vi "Horizontal Panel Example.vi"() -> ()   [LabVIEW 2016, in "PanelExample.lvclass"]
uses:
  PanelExample.lvclass
  PanelObject/PanelObject.lvclass
  <vilib>/Utility/error.llb/DialogType.ctl
  PanelDataNode/PanelDataNode.lvclass
  PanelDataNode/PanelDataNode.lvclass/PanelDataNode.ctl
  PanelDataNode/Split Mode.ctl
  QueueManager.llb/CreatQueue.vi
  QueueManager.llb/Remove.vi
  QueueManager.llb/Destroy.vi
  QueueManager.llb/Insert.vi
panel:
  in  "Node*":refnum<data-value>
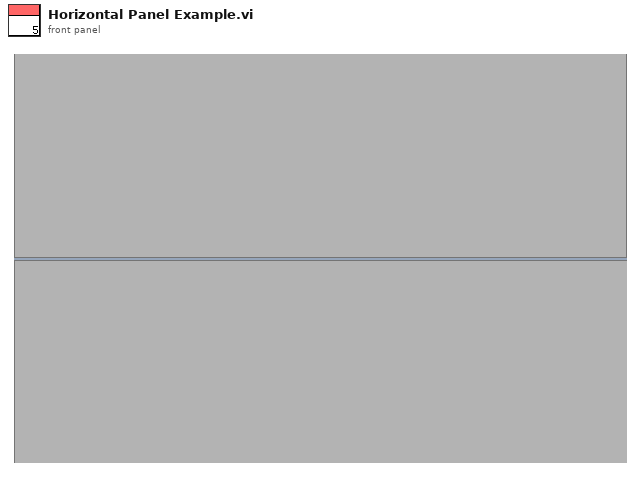
[diagram p1: front panel]
types:
  T1 = cluster{"error":errorcluster, "Event":string, "Data":variant, "Q_Local":string, "Caller":string, "Q_Root":string}
  T2 = typedef "PanelDataNode.lvclass/Split Mode.ctl" = enum16{"Horizontal(up)", "Vertical(left)", "Horizontal(down)", "Vertical(right)"}
  T3 = typedef "DialogType.ctl" = u16
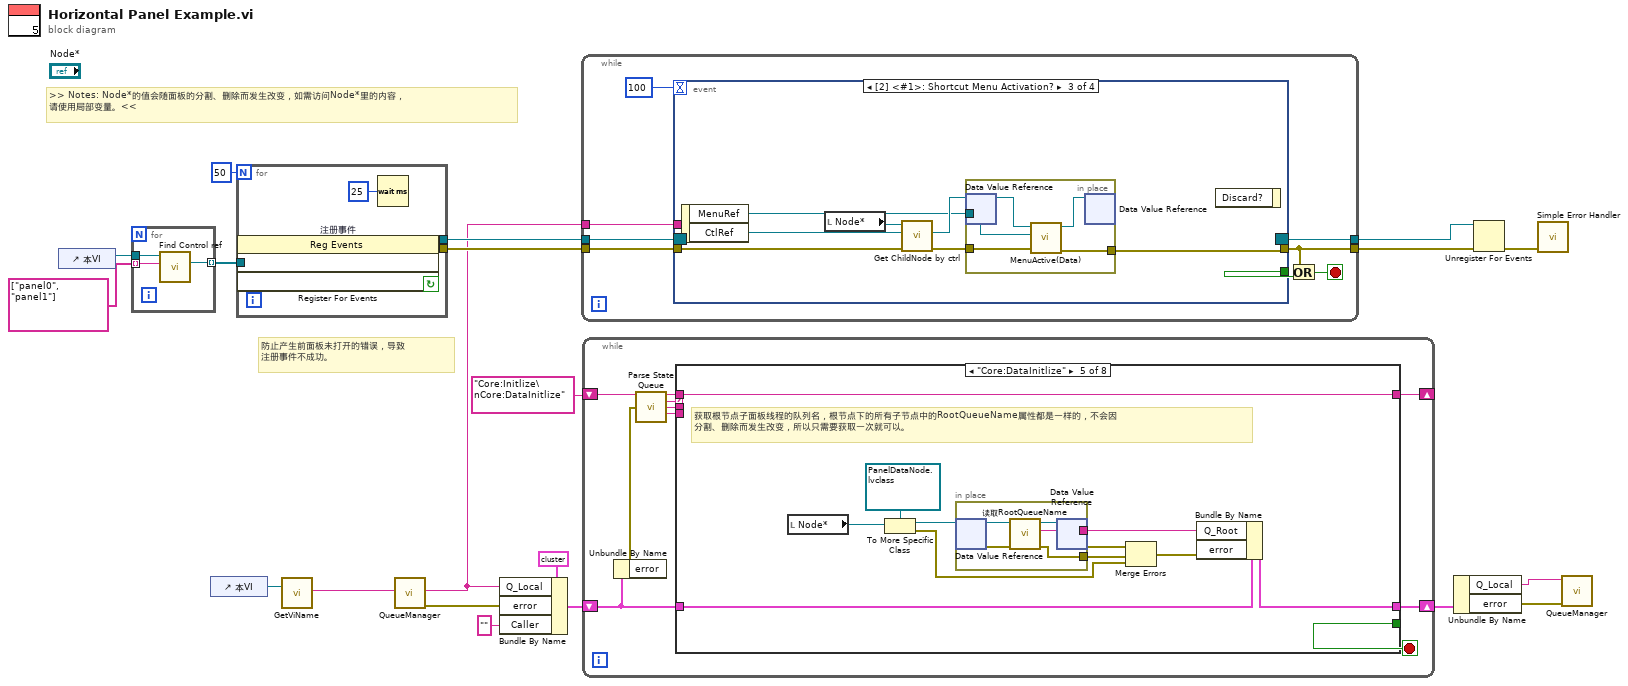
[diagram p0: block diagram]
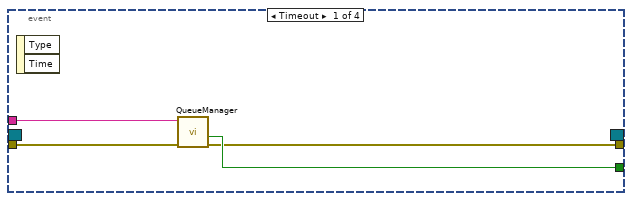
[diagram p2: hidden frame]
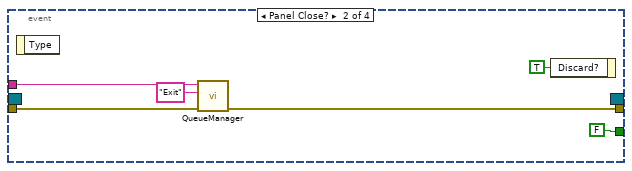
[diagram p3: hidden frame]
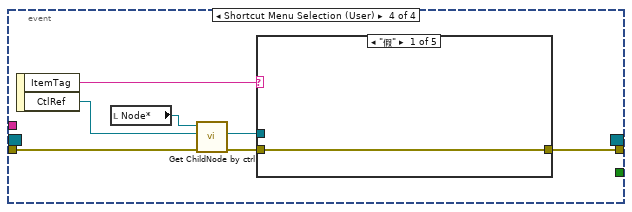
[diagram p4: hidden frame]
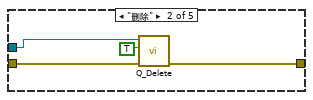
[diagram p5: hidden frame]
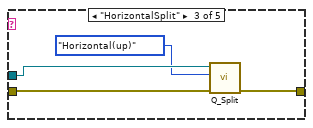
[diagram p6: hidden frame]
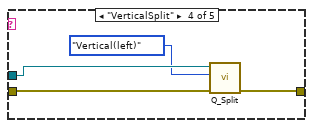
[diagram p7: hidden frame]
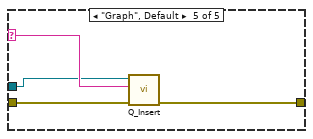
[diagram p8: hidden frame]
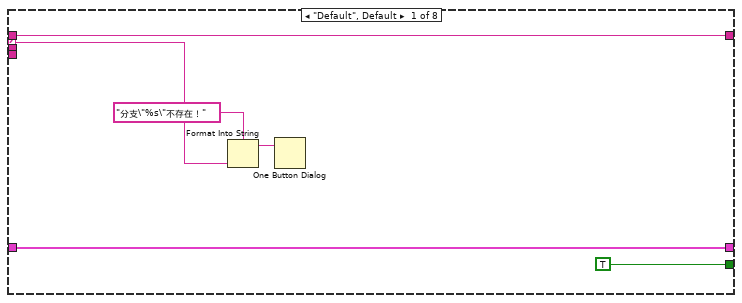
[diagram p9: hidden frame]
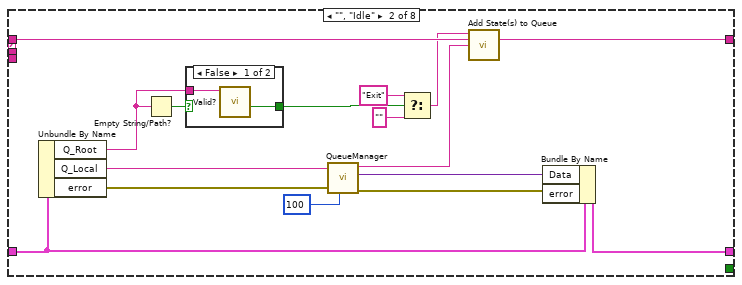
[diagram p10: hidden frame]
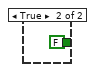
[diagram p11: hidden frame]
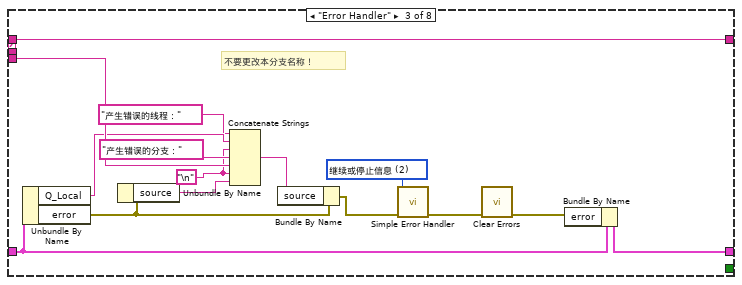
[diagram p12: hidden frame]
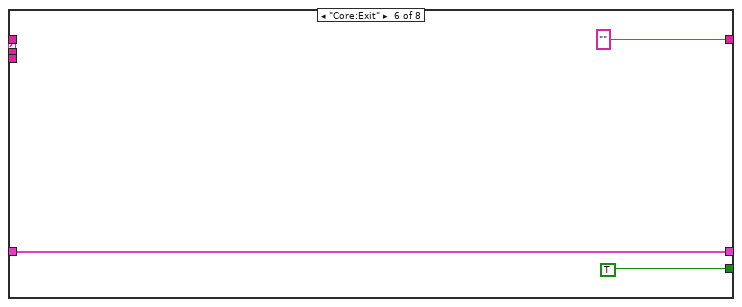
[diagram p14: hidden frame]
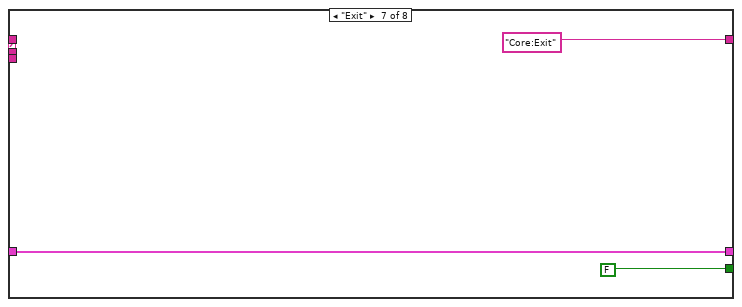
[diagram p15: hidden frame]
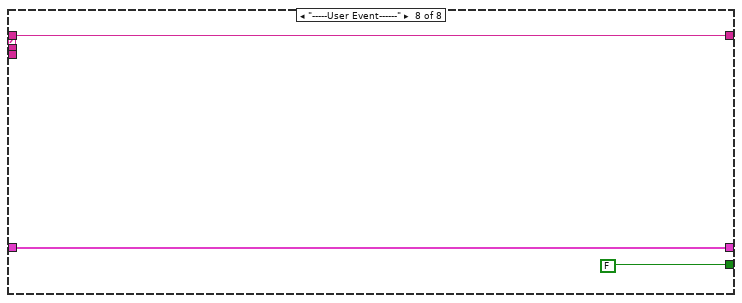
[diagram p16: hidden frame]
diagram:
  # ">> Notes: Node*的值会随面板的分割、删除而发生改变，如需访问Node*里的内容，\n请使用局部变量。<<"
  # "防止产生前面板未打开的错误，导致\n注册事件不成功。"
  n1 = control-ref of="本VI"() -> (w2:refnum<vi>)
  n2 = for {
    tunnel: w2 -> [w22]
    tunnel: string[] ["panel0", "panel1"] -> [w21] mode=indexing
    tunnel: [w20] -> w7 mode=indexing
    n3 = call "Find Control ref.vi"("control name"=w21, "panelvi*"=w22) -> ("ctrl*"=w20:refnum<vi>)  [unwired: 7 in, 2 out]
  }
  n4 = control-ref of="本VI"() -> (w12:refnum<vi>)
  n5 = for {
    N: 50 -> [_]
    tunnel: [w24] -> w10
    tunnel: [w26] -> w9
    tunnel: w7 -> [w25]
    stop <- w24 continue-if-true
    n6 = register-events "注册事件"(w25, w25) -> (reference out=w26:refnum<event-registration>, error out=w24:errorcluster)  [unwired: 2 in]
    n7 = Wait (ms)(milliseconds to wait=u32 25 ("等待时间（毫秒）")) -> ()  [unwired: 1 out]
  }
  n8 = call "GetViName.vi"("VI*"=w12) -> ("VI Name"=w8:string)  [unwired: 9 in, 1 out]
  n9 = call-poly "QueueManager.vi"("QueueName"=w8) -> ("error out"=w11:errorcluster)  [unwired: 9 in, 1 out]
  n10 = Bundle By Name(cluster=T1 {"error"={"status"=FALSE, "code"=0, "source"=""}, "Event"="", "Data"=variant, "Q_Local"="", "Caller"="", "Q_Root"=""} ("TmpData"), "Q_Local"=w8, "error"=w11, "Caller"="") -> (w15:T1)
  n11 = while {
    tunnel: w10 -> [w28]
    tunnel: w8 -> [w34]
    tunnel: [w31] -> w5
    tunnel: w9 -> [w29]
    tunnel: [w27] -> w3
    stop <- w32 stop-if-true
    n12 = event shown="[2] <#1>: Shortcut Menu Activation?" {
      selector: w29 -> [_ _ _ _]
      dyn-events: [_ _ _ _] -> w27
      timeout: 100 -> [_ _ _ _]
      tunnel: [w36 FALSE _ _] -> w33
      tunnel: w34 -> [w38 w43 _ _]
      tunnel: w28 -> [w37 w42 w48 w62]
      tunnel: [w35 w41 w46 w60] -> w31
      event Timeout {
        n13 = event-data() -> ()  [unwired: 1 in, 2 out]
        n14 = call-poly "QueueManager.vi"("error in (no error)"=w37, "Queue Name(unamed)"=w38) -> ("error out"=w35:errorcluster, "Not Exist?"=w36:bool)  [unwired: 8 in]
      }
      event Panel Close? {
        n15 = event-data() -> ()  [unwired: 1 in, 1 out]
        n16 = call-poly "QueueManager.vi"("error in"=w42, "Event"="Exit", "QueueName"=w43) -> ("error out"=w41:errorcluster)  [unwired: 7 in, 1 out]
        n17 = event-data("Discard?"=TRUE ("放弃？")) -> ()  [unwired: 1 in, 1 out]
      }
      event Shortcut Menu Activation? {
        n18 = event-data() -> ("MenuRef"=w45:refnum<k9>, "CtlRef"=w49:refnum<vi>)  [unwired: 1 in]
        n19 = local read "Node*"() -> (w50:refnum<data-value>)
        n20 = call "Get ChildNode by ctrl.vi"("error in (no error)"=w48, "ctr*"=w49, "Node*"=w50) -> ("error out"=w47:errorcluster, "ChildNode*"=w51:refnum<data-value>)  [unwired: 7 in]
        n21 = in-place {
          in-place-border: w45 -> [w55]
          in-place-border: w47 -> [w53]
          in-place-border: [w52] -> w46
          n22 = in-place-dvr #1(w51) -> (w56:refnum<class "PanelDataNode.lvclass">)  [unwired: 1 out]
          n23 = call-dynamic "MenuActive(Data).vi"("error in"=w53, "Menu Reference in"=w55, "PanelDataNode in"=w56) -> ("error out"=w52:errorcluster, "PanelDataNode out"=w54:refnum<class "PanelDataNode.lvclass">)  [unwired: 6 in, 1 out]
          n24 = in-place-dvr #1(w54) -> ()  [unwired: 2 out]
        }
        n25 = event-data() -> ()  [unwired: 2 in, 1 out]
      }
      event Shortcut Menu Selection (User) {
        n26 = event-data() -> ("ItemTag"=w59:string, "CtlRef"=w63:refnum<vi>)  [unwired: 1 in]
        n27 = local read "Node*"() -> (w57:refnum<data-value>)
        n28 = call "Get ChildNode by ctrl.vi"("error in (no error)"=w62, "ctr*"=w63, "Node*"=w57) -> ("error out"=w61:errorcluster, "ChildNode*"=w58:refnum<data-value>)  [unwired: 7 in]
        n29 = case shown="\"假\"" w59 {
          selector: w59 -> [_ _ _ _ w80]
          tunnel: w61 -> [w64 w67 w72 w76 w79]
          tunnel: [w64 w66 w71 w75 w77] -> w60
          tunnel: w58 -> [_ w65 w70 w74 w78]
          frame "假" {
          }
          frame "删除" {
            n30 = call "Q_Delete.vi"("error in"=w67, "CloseVI?(T)"=TRUE, "ChildNode*"=w65) -> ("error out"=w66:errorcluster)  [unwired: 8 in]
          }
          frame "HorizontalSplit" {
            n31 = call "Q_Split.vi"("error in"=w72, "Split Mode"=Split_Mode."Horizontal(up)", "ChildNode*"=w70) -> ("error out"=w71:errorcluster)  [unwired: 8 in]
          }
          frame "VerticalSplit" {
            n32 = call "Q_Split.vi"("error in"=w76, "Split Mode"=Split_Mode."Vertical(left)", "ChildNode*"=w74) -> ("error out"=w75:errorcluster)  [unwired: 8 in]
          }
          frame "Graph", Default {
            n33 = call "Q_Insert.vi"("error in"=w79, "Vi Alias"=w80, "ChildNode*"=w78) -> ("error out"=w77:errorcluster)  [unwired: 8 in]
          }
        }
      }
    }
    n34 = Or(x=w31, y=w33) -> (x .or. y?=w32:bool)
  }
  n35 = while {
    shift-right: [w84] -> w17
    shift-left: w15 -> [w85]
    shift-right: [w83] -> _
    shift-left: "Core:Initlize\nCore:DataInitlize" -> [w90]
    stop <- w87 stop-if-true
    n36 = Unbundle By Name(w85) -> ("error"=w86:errorcluster)
    n37 = call "Parse State Queue.vi"("State Queue"=w90, "Error In (no error)"=w86) -> ("Remaining States"=w89:string, "Current State"=w88:string, "Arguments"=w82:string, "PreState"=w81:string)  [unwired: 10 in]
    n38 = case shown="\"Core:DataInitlize\"" w88 {
      selector: w88 -> [w94 _ _ _ _ _ _ _]
      tunnel: w89 -> [w95 w109 w130 w132 w143 _ _ w155]
      tunnel: w82 -> [_ _ _ _ _ _ _ _]
      tunnel: [TRUE _ _ _ _ TRUE FALSE FALSE] -> w87
      tunnel: w85 -> [w96 w106 w127 w131 w139 w150 w153 w156]
      tunnel: [w96 w111 w126 w131 w138 w150 w153 w156] -> w84
      tunnel: [w95 w108 w130 w132 w143 "" ("Remaining States") "Core:Exit" ("Remaining States") w155] -> w83
      tunnel: w81 -> [_ _ w124 _ _ _ _ _]
      frame "Default", Default {
        n39 = Format Into String(format string="分支\"%s\"不存在！" ("格式字符串"), w94) -> (resulting string=w93:string)  [unwired: 2 in, 1 out]
        n40 = One Button Dialog(message=w93) -> ()  [unwired: 1 in, 1 out]
      }
      frame "", "Idle" {
        n41 = Unbundle By Name(w106) -> ("Q_Root"=w100:string, "Q_Local"=w105:string, "error"=w104:errorcluster)
        n42 = Empty String/Path?(string/path=w100) -> (empty?=w103:bool)
        n43 = case shown="False" w103 {
          tunnel: [w114 FALSE ("Not Exist?")] -> w102
          tunnel: w100 -> [w113 _]
          frame False {
            n44 = call "Valid?.vi"("Queue Name(unamed)"=w113) -> ("Not Exist?"=w114:bool)  [unwired: 9 in, 1 out]
          }
          frame True {
          }
        }
        n45 = call-poly "QueueManager.vi"("Time out(-1)"=100, "error in (no error)"=w104, "Queue Name"=w105) -> ("error out"=w112:errorcluster, "Data"=w110:variant, "Event"=w99:string)  [unwired: 5 in, 1 out]
        n46 = Select(t="Exit" ("Event"), s=w102, f="") -> (s? t:f=w97:string)
        n47 = call "Add State(s) to Queue.vi"("State(s) in Front (\"\")"=w97, "State(s) in (\"\")"=w109, "State(s) at Back (\"\")"=w99) -> ("States Out"=w108:string)  [unwired: 12 in]
        n48 = Bundle By Name(cluster=w106, "Data"=w110, "error"=w112) -> (w111:T1)
      }
      frame "Error Handler" {
        w117 = "\n"
        w125 = T3 2 items=["无对话框", "确定信息", "继续或停止信息", "确定信息＋警告", "继续/停止+警告"] ("type of dialog (OK msg:1)")
        # "不要更改本分支名称！"
        n49 = Unbundle By Name(w127) -> ("Q_Local"=w118:string, "error"=w120:errorcluster)
        n50 = Unbundle By Name(w120) -> ("source"=w122:string)
        n51 = Concatenate Strings("产生错误的线程：" ("字符串"), w118, w117, "产生错误的分支：" ("字符串"), w124, w117, w122) -> (w121:string)
        n52 = Bundle By Name(cluster=w120, "source"=w121) -> (w119:errorcluster)
        n53 = call <vilib>:"Simple Error Handler.vi"("type of dialog (OK msg:1)"=w125, "error in (no error)"=w119) -> ("error out"=w128:errorcluster)  [unwired: 3 in, 4 out]
        n54 = call <vilib>:"Clear Errors.vi"("error in (no error)"=w128) -> ("error out"=w129:errorcluster)  [unwired: 5 in, 1 out]
        n55 = Bundle By Name(cluster=w127, "error"=w129) -> (w126:T1)
      }
      frame "Core:Initlize" {
      }
      frame "Core:DataInitlize" {
        # "获取根节点子面板线程的队列名，根节点下的所有子节点中的RootQueueName属性都是一样的，不会因\n分割、删除而发生改变，所以只需要获取一次就可以。"
        n56 = local read "Node*"() -> (w140:refnum<data-value>)
        n57 = To More Specific Class(target class=refnum<data-value> refnum ("Node*"), reference=w140) -> (specific class reference=w142:refnum<data-value>, error out=w133:errorcluster)  [unwired: 1 in]
        n58 = in-place {
          in-place-border: [w145] -> w137
          in-place-border: [w144] -> w136
          n59 = in-place-dvr #2(w142) -> (w148:refnum<class "PanelDataNode.lvclass">, w146:errorcluster)
          n60 = call "读取RootQueueName.vi"("error in (no error)"=w146, "PanelDataNode输入"=w148) -> ("error out"=w144:errorcluster, "RootQueueName"=w145:string, "PanelDataNode输出"=w147:refnum<class "PanelDataNode.lvclass">)  [unwired: 7 in]
          n61 = in-place-dvr #2(w147) -> (w135:errorcluster)  [unwired: 1 out]
        }
        n62 = Merge Errors(w135, w136, w133) -> (w134:errorcluster)
        n63 = Bundle By Name(cluster=w139, "Q_Root"=w137, "error"=w134) -> (w138:T1)
      }
      frame "Core:Exit" {
      }
      frame "Exit" {
      }
      frame "-----User Event------" {
      }
    }
  }
  n64 = Unbundle By Name(w17) -> ("Q_Local"=w14:string, "error"=w18:errorcluster)
  n65 = Unregister For Events(event registration refnum=w3, error in=w5) -> (error out=w4:errorcluster)
  n66 = call <vilib>:"Simple Error Handler.vi"("error in (no error)"=w4) -> ()  [unwired: 4 in, 5 out]
  n67 = call-poly "QueueManager.vi"("error in (no error)"=w18, "QueeuName"=w14) -> ()  [unwired: 9 in, 1 out]
